vi "Actor Core.vi"(8 "error in":errorcluster, 11 "ATM Controller in":refnum<class "Sim Display Console Actor.lvclass">) -> (0 "error out":errorcluster, 3 "Actor out":refnum<class "Actor.lvclass">)   [LabVIEW 2019, in "Sim Display Console Actor.lvlib" / "Sim Display Console Actor.lvclass"]
doc: "(<B>Filename</B>: Actor Framework.lvlib:Actor.lvclass:Actor Core.vi)\n\nReceives messages to the actor, reacts to them, and initiates any error handling that may shut the actor down.\n\nDescendant classes may override this VI to append parallel tasks for the actor to complete while it handles messages. Overrides use the Call Parent Method node."
uses:
  Sim Display Console Actor.lvclass
  <vilib>/ActorFramework/Stop Msg/Stop Msg.lvclass
  <vilib>/ActorFramework/Actor/Actor.lvclass
  Display Console Actor/Display Console Actor/Display Console Actor.lvclass
  C:/Workspace/CLA/ATM AF 2nd/Display Console Actor/Display Console Actor/Display Console Actor.lvclass
  C:/Program Files (x86)/National Instruments/LabVIEW 2019/vi.lib/ActorFramework/Actor/Actor.lvclass
  Transaction -Enum.ctl
panel:
  out "Message":string
  out "Transaction":T1=enum."Balance Inquiry"
  out "Card Read":bool
  # "[Covers: UI3] \n\n[Covers: UI3C]"
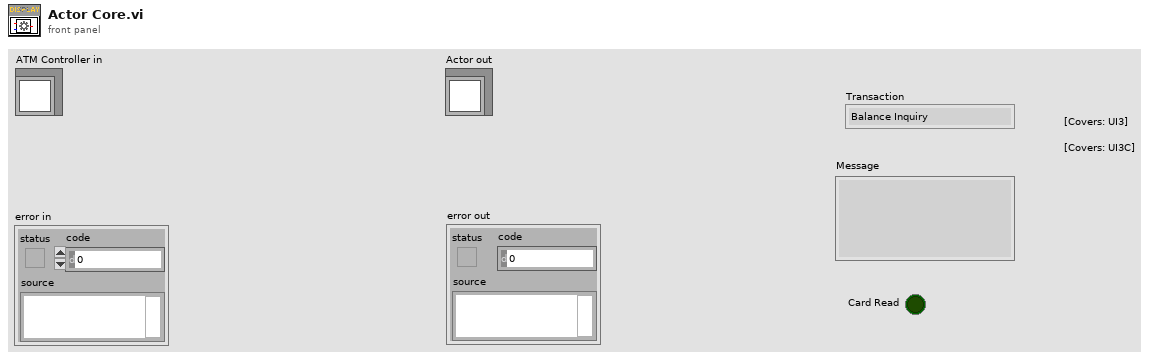
[diagram p1: front panel]
types:
  T1 = typedef "Sim Display Console Actor.lvlib/Sim Display Console Actor.lvclass/Transaction -Enum.ctl" = enum16{"", "Balance Inquiry", "Deposit", "Withdrawal", "Fast Cash $50", "New Transaction", "Terminate Session"}
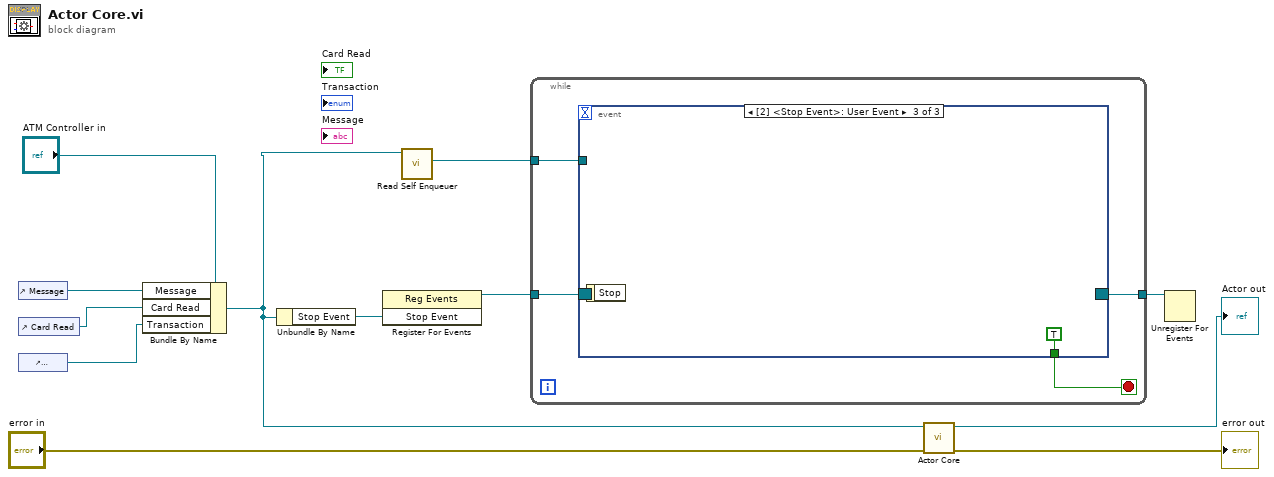
[diagram p0: block diagram]
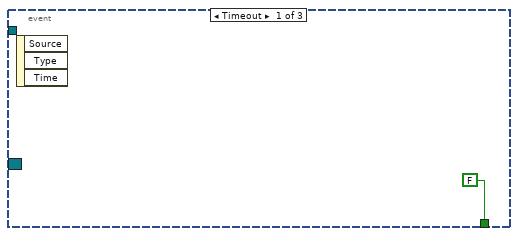
[diagram p2: hidden frame]
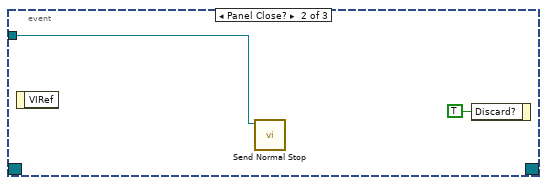
[diagram p3: hidden frame]
diagram:
  n1 = control-ref of="Message"() -> (w3:refnum<vi>)
  n2 = control-ref of="Card Read"() -> (w2:refnum<vi>)
  n3 = control-ref of="Transaction"() -> (w1:refnum<vi>)
  n4 = Bundle By Name(cluster="ATM Controller in", "Message"=w3, "Card Read"=w2, "Transaction"=w1) -> (w4:refnum<class "Sim Display Console Actor.lvclass">)
  n5 = Unbundle By Name(w4) -> ("Stop Event"=w9:refnum<user-event>)
  n6 = register-events(w9) -> (reference out=w8:refnum<event-registration>)  [unwired: 2 in, 1 out]
  n7 = call <vilib>:"Read Self Enqueuer.vi"("Actor"=w4) -> ("Self Enqueuer"=w6:refnum<class "Message Enqueuer.lvclass">)  [unwired: 10 in]
  n8 = while {
    tunnel: w8 -> [w15]
    tunnel: [w14] -> w7
    tunnel: w6 -> [w13]
    stop <- w16 stop-if-true
    n9 = event shown="[2] <Stop Event>: User Event" {
      selector: w15 -> [_ _ _]
      dyn-events: [_ _ _] -> w14
      timeout: _ -> [_ _ _]
      tunnel: [FALSE _ TRUE] -> w16
      tunnel: w13 -> [_ w19 _]
      event Timeout {
        n10 = event-data() -> ()  [unwired: 1 in, 3 out]
      }
      event Panel Close? {
        n11 = event-data() -> ()  [unwired: 1 in, 1 out]
        n12 = call <vilib>:"Send Normal Stop.vi"("Message Enqueuer"=w19) -> ()  [unwired: 10 in, 1 out]
        n13 = event-data("Discard?"=TRUE) -> ()  [unwired: 1 in, 1 out]
      }
      event User Event {
        n14 = event-data() -> ()  [unwired: 1 in, 1 out]
      }
    }
  }
  n15 = call-parent "Actor Core.vi"("error in"="error in", "Actor in"=w4) -> ("error out"=→"error out":errorcluster, "Actor out"=→"Actor out":refnum<class "Actor.lvclass">)  [unwired: 8 in]
  n16 = Unregister For Events(event registration refnum=w7) -> ()  [unwired: 1 in, 1 out]
